vi "Send Query.vi"(8 "error in (no error)":errorcluster, 10 "query string":string, 11 "VISA resource name":refnum<visa-resource-name>="COM1") -> (0 "error out":errorcluster, 1 "read buffer":string, 2 "query output":string, 3 "VISA resource name out":refnum<visa-resource-name>)   [LabVIEW 2017]
panel:
  in  "Bytes Count":u32=1024
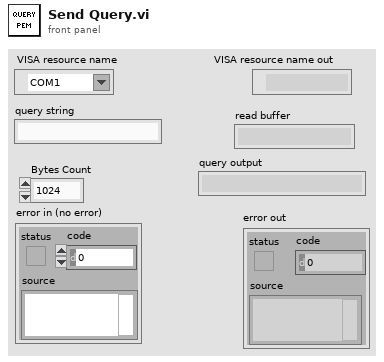
[diagram p1: front panel]
types:
  T1 = typedef "Semaphore RefNum" = refnum<k1>
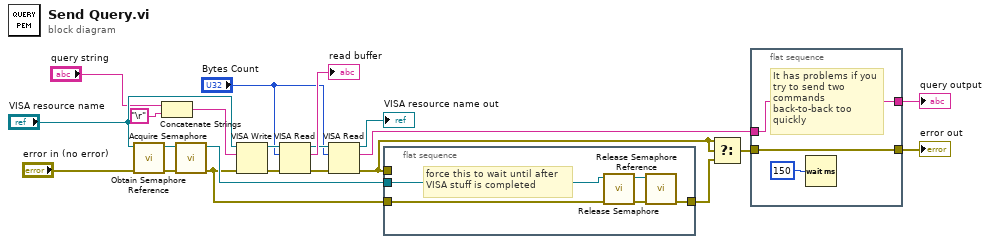
[diagram p0: block diagram]
diagram:
  n1 = call <vilib>:"Obtain Semaphore Reference.vi"("error in (no error)"="error in (no error)", "name (unnamed)"="VISA resource name") -> ("error out"=w19:errorcluster, "semaphore"=w20:T1)  [unwired: 1 in, 3 out]
  n2 = Concatenate Strings("query string", "\r") -> (w1:string)
  n3 = call <vilib>:"Acquire Semaphore.vi"("error in (no error)"=w19, "semaphore"=w20) -> ("error out"=w14:errorcluster, "semaphore out"=w17:T1)  [unwired: 1 in, 3 out]
  n4 = VISA Write(VISA resource name="VISA resource name", write buffer=w1, error in (no error)=w14) -> (VISA resource name out=w22:refnum<visa-resource-name>, error out=w21:errorcluster)  [unwired: 1 out]
  n5 = VISA Read(VISA resource name=w22, byte count="Bytes Count", error in (no error)=w21) -> (VISA resource name out=w12:refnum<visa-resource-name>, read buffer=→"read buffer":string, error out=w11:errorcluster)  [unwired: 1 out]
  n6 = VISA Read(VISA resource name=w12, byte count="Bytes Count", error in (no error)=w11) -> (VISA resource name out=→"VISA resource name out":refnum<visa-resource-name>, read buffer=w8:string, error out=w5:errorcluster)  [unwired: 1 out]
  n7 = flat-sequence {
    tunnel: w17 -> [w27]
    tunnel: [w24] -> w15
    tunnel: w14 -> [w23]
    tunnel: w5 -> [_]
    frame #0 {
      # "force this to wait until after \nVISA stuff is completed"
      n8 = call <vilib>:"Release Semaphore.vi"("error in (no error)"=w23, "semaphore"=w27) -> ("error out"=w25:errorcluster, "semaphore out"=w26:T1)  [unwired: 4 out]
      n9 = call <vilib>:"Release Semaphore Reference.vi"("error in (no error)"=w25, "semaphore"=w26) -> ("error out"=w24:errorcluster)  [unwired: 9 out]
    }
  }
  n10 = Select(t=w5, s=w5, f=w15) -> (s? t:f=w9:errorcluster)
  n11 = flat-sequence {
    tunnel: [w30] -> w10
    tunnel: w9 -> [w30]
    tunnel: w8 -> [w29]
    tunnel: [w29] -> w7
    frame #0 {
      # "It has problems if you try to send two commands back-to-back too quickly"
      n12 = Wait (ms)(milliseconds to wait=u32 150) -> ()  [unwired: 1 out]
    }
  }
  "error out" <- w10
  "query output" <- w7
